vi "All results calculation.vi"(8 "频率配置":i32, 9 "平均混响时间T2":dbl[](array[numeric]), 10 "平均混响时间T1":dbl[](array[numeric])) -> (0 "分立吸声体吸声量Aobj":dbl[](array[numeric]), 1 "试件吸声量AT":dbl[](array[numeric]), 2 "混响室吸声量A2":dbl[](array[numeric]), 3 "混响室吸声量A1":dbl[](array[numeric]), 4 "吸声系数αs":dbl[](array[numeric]), 5 "rowhead":string[](array[string])=["A1", "A2", "AT", "Aobj", "αs"])   [LabVIEW 2020]
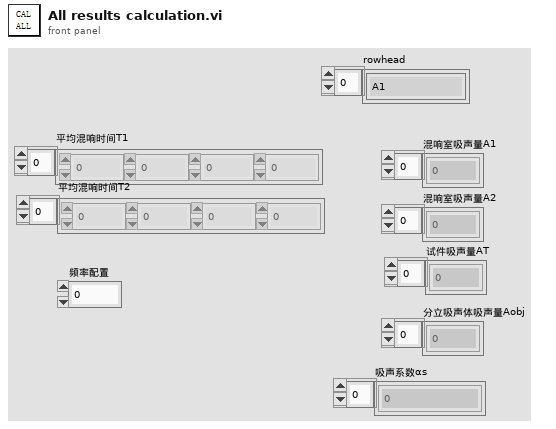
[diagram p1: front panel]
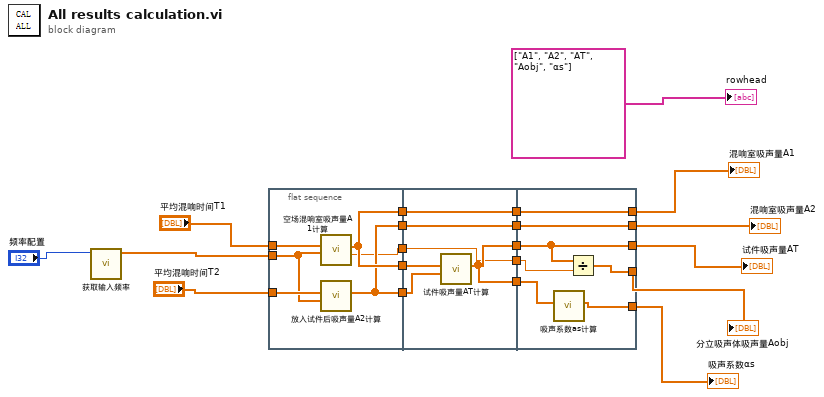
[diagram p0: block diagram]
diagram:
  n1 = call "获取输入频率.vi"("频率配置"="频率配置") -> ("频率"=w1:dbl[])  [unwired: 10 in]
  n2 = flat-sequence {
    tunnel: "平均混响时间T1" -> [w26]
    tunnel: "平均混响时间T2" -> [w25]
    tunnel: [w24] -> w18
    tunnel: [w23] -> w17
    tunnel: [w24] -> w13
    tunnel: [w23] -> w11
    tunnel: [w22] -> w4
    tunnel: w1 -> [w21]
    tunnel: w18 -> [w32]
    tunnel: w17 -> [w31]
    tunnel: [w28] -> w16
    tunnel: [w30] -> w14
    tunnel: w13 -> [w30]
    tunnel: [w29] -> w12
    tunnel: w11 -> [w29]
    tunnel: [w28] -> w10
    tunnel: [w27] -> w5
    tunnel: w4 -> [w27]
    tunnel: w16 -> [w39]
    tunnel: [w38] -> w15
    tunnel: [w37] -> w9
    tunnel: w14 -> [w37]
    tunnel: [w36] -> w8
    tunnel: w12 -> [w36]
    tunnel: [w35] -> w7
    tunnel: w10 -> [w35]
    tunnel: [w34] -> w6
    tunnel: w5 -> [w33]
    frame #0 {
      n3 = call "空场混响室吸声量A1计算.vi"("频率"=w21, "平均混响时间T1"=w26) -> ("分立吸声体个数，n"=w22:dbl, "混响室吸声量A1"=w24:dbl[])  [unwired: 8 in]
      n4 = call "放入试件后吸声量A2计算.vi"("频率"=w21, "平均混响时间T2"=w25) -> ("混响室吸声量A2"=w23:dbl[])  [unwired: 9 in]
    }
    frame #1 {
      n5 = call "试件吸声量AT计算.vi"("混响室吸声量A1"=w32, "混响室吸声量A2"=w31) -> ("试件吸声量AT"=w28:dbl[])  [unwired: 7 in]
    }
    frame #2 {
      n6 = call "吸声系数as计算.vi"("试件吸声量AT"=w39) -> ("吸声系数as"=w38:dbl[])  [unwired: 10 in]
      n7 = Divide(x=w35, y=w33) -> (x/y=w34:dbl[])
    }
  }
  "吸声系数αs" <- w15
  "混响室吸声量A1" <- w9
  "混响室吸声量A2" <- w8
  "试件吸声量AT" <- w7
  "分立吸声体吸声量Aobj" <- w6
  "rowhead" <- string[] ["A1", "A2", "AT", "Aobj", "αs"]
